vi "GetDeviceInfo.vi"   [LabVIEW 2011, in "MvCameraControl.lvlib"]
uses:
  MvCameraControl.lvlib
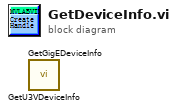
[diagram p0: block diagram]
diagram:
  n1 = call "GetU3VDeviceInfo.vi"() -> ()  [unwired: 8 in, 3 out]
  n2 = call "GetGigEDeviceInfo.vi"() -> ()  [unwired: 8 in, 3 out]
